vi "Sort 2D Num Array DESCENDING - Bubble Sort.vi"(8 "Column to Sort By":i32=1, 10 "Input 2D Array":i32[][](array[numeric])=[[0, 0, 0], [0, 0, 0], [0, 0, 0], [0, 0, 0], [0, 0, 0], [0, 0, 0], [0, 0, 0], [0, 0, 0]]) -> (1 "Sorted Array":i32[][](array[numeric]))   [LabVIEW 2010]
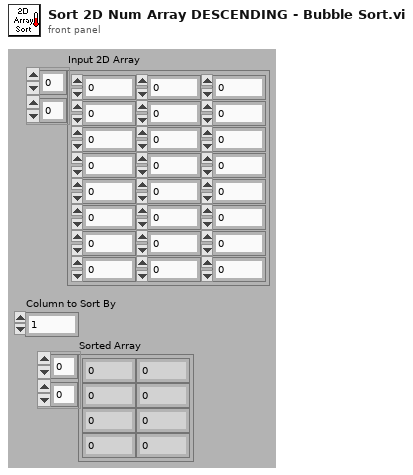
[diagram p1: front panel]
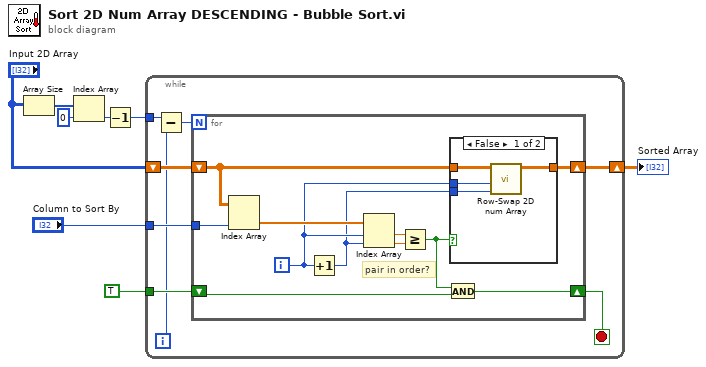
[diagram p0: block diagram]
diagram:
  n1 = Array Size(array="Input 2D Array") -> (size(s)=w7:i32[])
  n2 = Index Array(array=w7, index=0) -> (element=w4:i32)
  n3 = Decrement(x=w4) -> (x-1=w8:i32)
  n4 = while {
    tunnel: w8 -> [w16]
    tunnel: "Column to Sort By" -> [w13]
    tunnel: TRUE ("x <= y?") -> [w12]
    shift-right: [w15] -> w6
    shift-left: "Input 2D Array" -> [w14]
    i -> [w9]
    stop <- w11 stop-if-true
    n5 = Subtract(x=w16, y=w9) -> (x-y=w10:i32)
    n6 = for {
      N: w10 -> [_]
      shift-right: [w17] -> w15
      shift-left: w14 -> [w27]
      tunnel: w13 -> [w26]
      shift-right: [w22] -> w11
      shift-left: w12 -> [w20]
      i -> [w19]
      # "pair in order?"
      n7 = Index Array "Index Array"(array=w27, index (col)=w26) -> (element=w25:dbl[])  [unwired: 1 in]
      n8 = Increment(x=w19) -> (x+1=w18:i32)
      n9 = Index Array "Index Array"(array=w25, index #1=w19, index #2=w18) -> (element #1=w23:dbl, element #2=w24:dbl)
      n10 = Greater Or Equal?(x=w23, y=w24) -> (x >= y?=w21:bool)
      n11 = And(x=w21, y=w20) -> (x .and. y?=w22:bool)
      n12 = case shown="False" w21 {
        tunnel: w27 -> [w31 w32]
        tunnel: [w30 w32] -> w17
        tunnel: w19 -> [w29 _]
        tunnel: w18 -> [w28 _]
        frame False {
          n13 = call "Row-Swap 2D num Array.vi"("Index b"=w28, "Index a"=w29, "row-swapped array"=w31) -> ("row-swapped array"=w30:dbl[][])  [unwired: 8 in]
        }
        frame True {
        }
      }
    }
  }
  "Sorted Array" <- w6
